vi "command_get_current_position.vi"(8 "error in (no error)":errorcluster, 11 "StageMH110930Scientifica in":refnum<class "StageMMS2015ASIfromScientifica.lvclass">) -> (0 "error out":errorcluster, 2 "current position":refnum<class "SpaceVector.lvclass">, 3 "StageMH110930Scientifica out":refnum<class "StageMMS2015ASIfromScientifica.lvclass">)   [LabVIEW 2010, in "StageMMS2015ASIfromScientifica.lvclass"]
uses:
  StageMMS2015ASIfromScientifica.lvclass
  common/classes/SpaceVector/SpaceVector/SpaceVector.lvclass
  common/classes/ErrorController/ErrorController/class_data.vi
  common/classes/ErrorController/ErrorController/ErrorController.lvclass
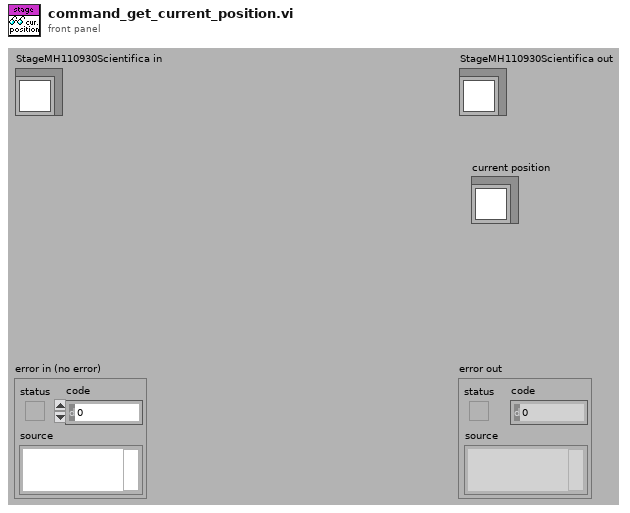
[diagram p1: front panel]
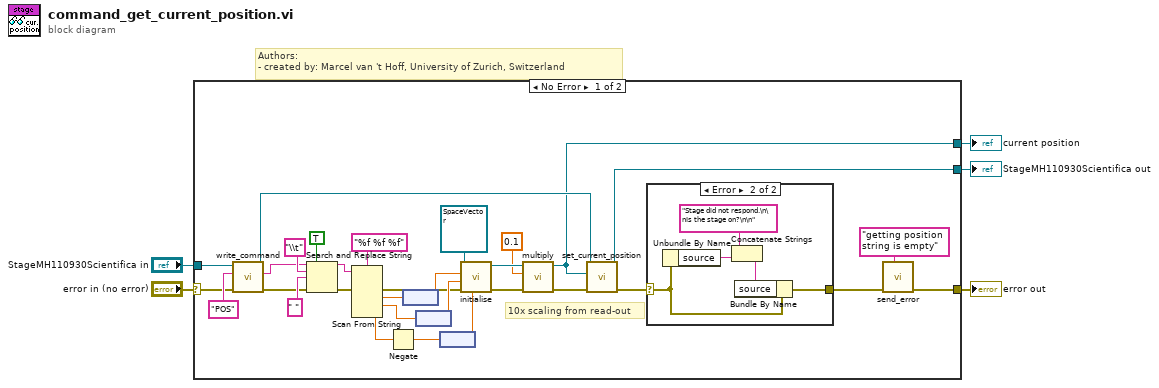
[diagram p0: block diagram]
diagram:
  # "Authors: \n- created by: Marcel van 't Hoff, University of Zurich, Switzerland"
  n1 = case shown="No Error" "error in (no error)" {
    selector: "error in (no error)" -> [w32 w44]
    tunnel: [w10 w44] -> w4
    tunnel: [w33 w43] -> w2
    tunnel: "StageMH110930Scientifica in" -> [w36 w43]
    tunnel: [w14 _] -> w1
    frame No Error {
      # "10x scaling from read-out"
      n2 = call-dynamic "write_command.vi"("error in (no error)"=w32, "string to write"="POS", "StageMH110930Scientifica in"=w36) -> ("error out"=w18:errorcluster, "read string"=w17:string, "StageMH110930Scientifica out"=w34:refnum<class "StageMMS2015ASIfromScientifica.lvclass">)  [unwired: 5 in, 1 out]
      n3 = Search and Replace String(replace all?=TRUE ("replace all? (F)"), input string=w17, search string="\\t", replace string=" " ("replace string (\"\")"), error in=w18) -> (result string=w20:string, error out=w16:errorcluster)  [unwired: 3 in, 2 out]
      n4 = Scan From String(format string="%f %f %f", input string=w20, error in=w16) -> (error out=w23:errorcluster, output 1=w30:dbl, output 2=w29:dbl, output 3=w28:dbl)  [unwired: 1 in, 5 out]
      n5 = Negate(x=w28) -> (-x=w6:dbl)
      n6 = node(w30) -> (w27:dbl[unit])
      n7 = node(w29) -> (w26:dbl[unit])
      n8 = node(w6) -> (w25:dbl[unit])
      n9 = call "initialise.vi"("z"=w25, "error in (no error)"=w23, "y"=w26, "x"=w27, "SpaceVector in"=refnum<class "SpaceVector.lvclass"> refnum) -> ("error out"=w13:errorcluster, "SpaceVector out"=w15:refnum<class "SpaceVector.lvclass">)  [unwired: 5 out]
      n10 = call "multiply.vi"("error in (no error)"=w13, "factor"=0.1, "SpaceVector in"=w15) -> ("error out"=w12:errorcluster, "SpaceVector out"=w14:refnum<class "SpaceVector.lvclass">)  [unwired: 7 in]
      n11 = call-dynamic "set_current_position.vi"("error in (no error)"=w12, "current position"=w14, "DL090409StageScaffold.lvclass in"=w34) -> ("error out"=w8:errorcluster, "DL090409StageScaffold.lvclass out"=w33:refnum<class "StageMMS2015ASIfromScientifica.lvclass">)  [unwired: 7 out]
      n12 = case shown="Error" w8 {
        selector: w8 -> [w37 w42]
        tunnel: [w37 w41] -> w7
        frame No Error {
        }
        frame Error {
          n13 = Unbundle By Name(w42) -> ("source"=w39:string)
          n14 = Concatenate Strings("Stage did not respond.\n\nIs the stage on?\n\n" ("string"), w39) -> (w40:string)
          n15 = Bundle By Name(cluster=w42, "source"=w40) -> (w41:errorcluster)
        }
      }
      n16 = call "send_error.vi"("additional message"="getting position string is empty", "error in (no error)"=w7) -> ("error out"=w10:errorcluster)  [unwired: 9 in]
    }
    frame Error {
    }
  }
  "error out" <- w4
  "StageMH110930Scientifica out" <- w2
  "current position" <- w1
